vi "ConvertParameters.vi"(11 "ParameterDefs":T3[](array[typedef])) -> (3 "Parameters":T1[](array[typedef]))   [LabVIEW 2017, in "MessageGen.lvlib"]
uses:
  <vilib>/addons/InsightCM/MessageBus/CodeGen/MessageGen.lvlib
  <vilib>/addons/InsightCM/MessageBus/CodeGen/controls/ParameterDef.ctl
  <vilib>/addons/InsightCM/MessageBus/CodeGen/controls/Parameter.ctl
  <vilib>/addons/InsightCM/MessageBus/CodeGen/controls/ParameterType.ctl
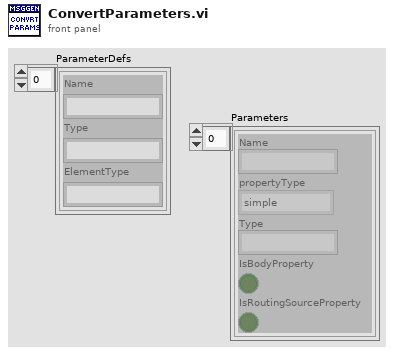
[diagram p1: front panel]
types:
  T1 = typedef "MessageGen.lvlib/Parameter.ctl" = cluster{"Name":string, "propertyType":T2, "Type":string, "IsBodyProperty":bool, "IsRoutingSourceProperty":bool}
  T2 = typedef "MessageGen.lvlib/ParameterType.ctl" = enum16{"simple", "bytearray", "dateTime", "list", "map", "object"}
  T3 = typedef "MessageGen.lvlib/ParameterDef.ctl" = cluster{"Name":string, "Type":string, "ElementType":string}
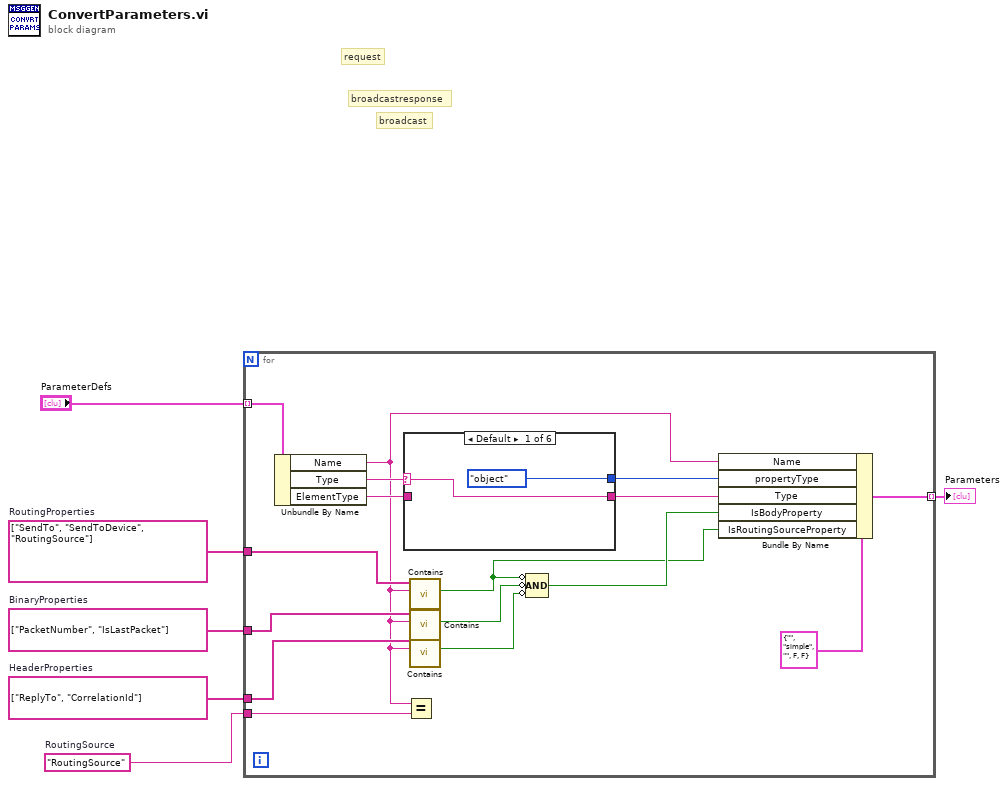
[diagram p0: block diagram]
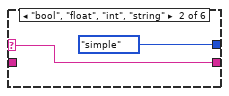
[diagram p2: hidden frame]
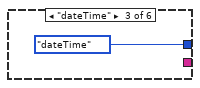
[diagram p3: hidden frame]
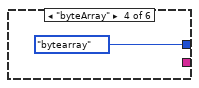
[diagram p4: hidden frame]
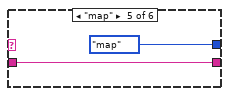
[diagram p5: hidden frame]
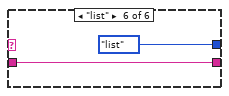
[diagram p6: hidden frame]
diagram:
  w2 = "RoutingSource"  # RoutingSource
  w3 = string[] ["ReplyTo", "CorrelationId"]  # HeaderProperties
  w4 = string[] ["PacketNumber", "IsLastPacket"]  # BinaryProperties
  w5 = string[] ["SendTo", "SendToDevice", "RoutingSource"]  # RoutingProperties
  # "broadcast"
  # "broadcastresponse"
  # "request"
  n1 = for {
    tunnel: "ParameterDefs" -> [w22] mode=indexing
    tunnel: w5 -> [w16]
    tunnel: w4 -> [w15]
    tunnel: w3 -> [w14]
    tunnel: w2 -> [w13]
    tunnel: [w8] -> w1 mode=indexing
    n2 = Unbundle By Name(w22) -> ("Name"=w12:string, "Type"=w21:string, "ElementType"=w20:string)
    n3 = case shown="Default" w21 {
      selector: w21 -> [w23 w25 _ _ _ _]
      tunnel: [ParameterType."object" ("propertyType") ParameterType."simple" ("propertyType") ParameterType."dateTime" ("propertyType") ParameterType."bytearray" ("propertyType") ParameterType."map" ("propertyType") ParameterType."list" ("propertyType")] -> w18
      tunnel: [w23 w25 _ _ w29 w31] -> w17
      tunnel: w20 -> [_ _ _ _ w29 w31]
      frame Default {
      }
      frame "bool", "float", "int", "string" {
      }
      frame "dateTime" {
      }
      frame "byteArray" {
      }
      frame "map" {
      }
      frame "list" {
      }
    }
    n4 = Equal?(x=w12, y=w13) -> ()  [unwired: 1 out]
    n5 = call <vilib>:"Contains.vi"("Item"=w12, "List"=w16) -> ("Contains"=w7:bool)  [unwired: 9 in]
    n6 = call <vilib>:"Contains.vi"("Item"=w12, "List"=w15) -> ("Contains"=w11:bool)  [unwired: 9 in]
    n7 = call <vilib>:"Contains.vi"("Item"=w12, "List"=w14) -> ("Contains"=w10:bool)  [unwired: 9 in]
    n8 = Compound Arithmetic op=AND(invert w7, invert w11, invert w10) -> (w9:bool)
    n9 = Bundle By Name(cluster=T1 {"Name"="", "propertyType"=enum."simple", "Type"="", "IsBodyProperty"=FALSE, "IsRoutingSourceProperty"=FALSE} ("Property"), "Name"=w12, "propertyType"=w18, "Type"=w17, "IsBodyProperty"=w9, "IsRoutingSourceProperty"=w7) -> (w8:T1)
  }
  "Parameters" <- w1
